vi "Read Peaks and Levels.vi"(0 "VISA resource name":refnum<visa-resource-name>, 5 "Enable Unbuffered Data (Enabled)":bool=TRUE, 11 "error in (no error)":errorcluster) -> (2 "Status":T2 {"Time Stamp" format="%#_20f"; "Operating Mode" items=["Stand-Alone", "Master", "End Slave", "Middle Slave"]; "Trigger Mode" items=["Untriggered", "Software Triggered", "Hardware Triggered"]; "Full Spectrum Radix" format="%b"}, 3 "Data Status":T3 {"Sub-Channel" items=["None", "1", "2", "3", "4"]; "Time Stamp" format="%#_20f"}, 4 "VISA resource name out":refnum<visa-resource-name>, 6 "Number of Sensors":u16[](array[numeric]), 8 "Amplitude (dBm)":i16[](array[numeric]), 10 "Peak Wavelengths (nm)":dbl[][](array[numeric]) format="%#_10g", 13 "Reserved":T1, 14 "Trigger Mode":u8(ring) items=["Untriggered", "Software Triggered", "Hardware Triggered"], 15 "error out":errorcluster)   [LabVIEW 2024, in "Micron Optics sm130.lvlib"]
doc: "Displays the peaks and levels. Peaks correspond to Peak Wavelengths in nm and Levels to Amplitudes in dBm."
uses:
  Micron Optics sm130.lvlib
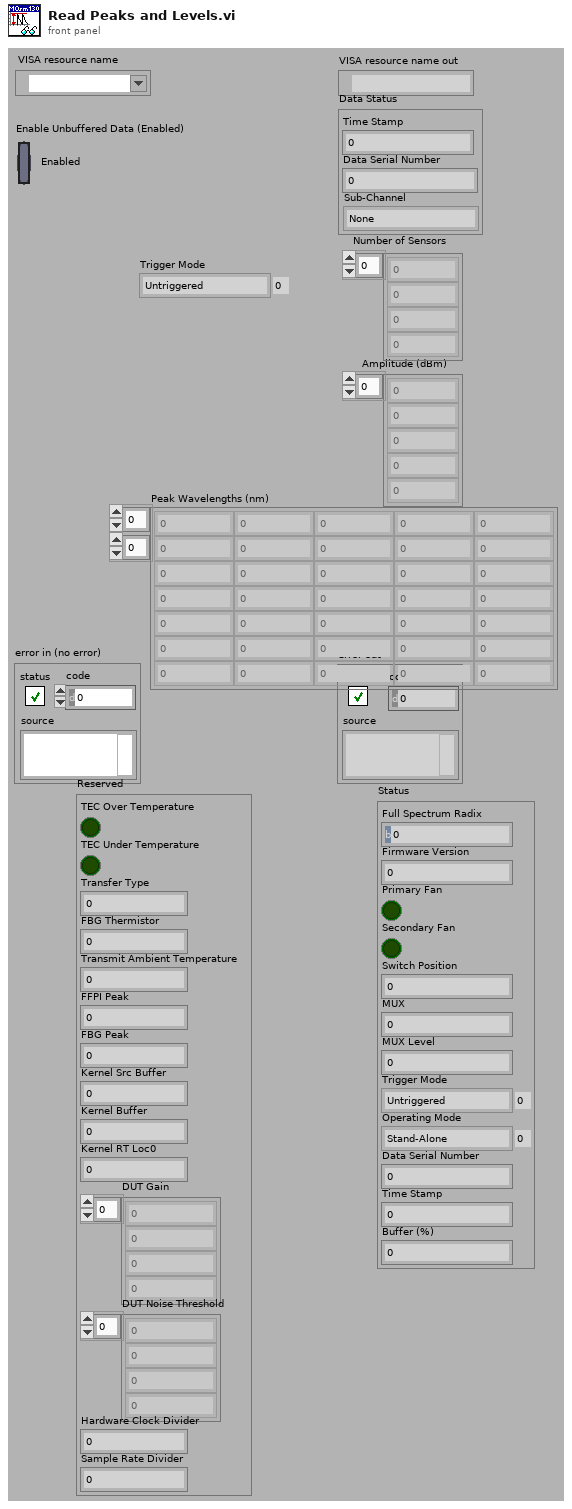
[diagram p1: front panel]
types:
  T1 = cluster{"Transmit Ambient Temperature":dbl, "FBG Thermistor":i16, "FFPI Peak":u16, "FBG Peak":dbl, "Kernel Src Buffer":u16, "Kernel Buffer":u16, "Kernel RT Loc0":u32, "DUT Gain":u16[], "DUT Noise Threshold":u16[], "Hardware Clock Divider":u16, "Sample Rate Divider":u16, "TEC Over Temperature":bool, "TEC Under Temperature":bool, "Transfer Type":u8}
  T2 = cluster{"Full Spectrum Radix":u8, "Firmware Version":u8, "Primary Fan":bool, "Secondary Fan":bool, "Switch Position":u8, "MUX":u8, "Trigger Mode":u8, "Operating Mode":u8, "Data Serial Number":u32, "Time Stamp":dbl, "Buffer (%)":u8, "MUX Level":u8}
  T3 = cluster{"Data Serial Number":u32, "Time Stamp":dbl, "Sub-Channel":u8}
  T4 = cluster{"Data Serial Number":u32, "Time Stamp":dbl, "Switch Position":u8}
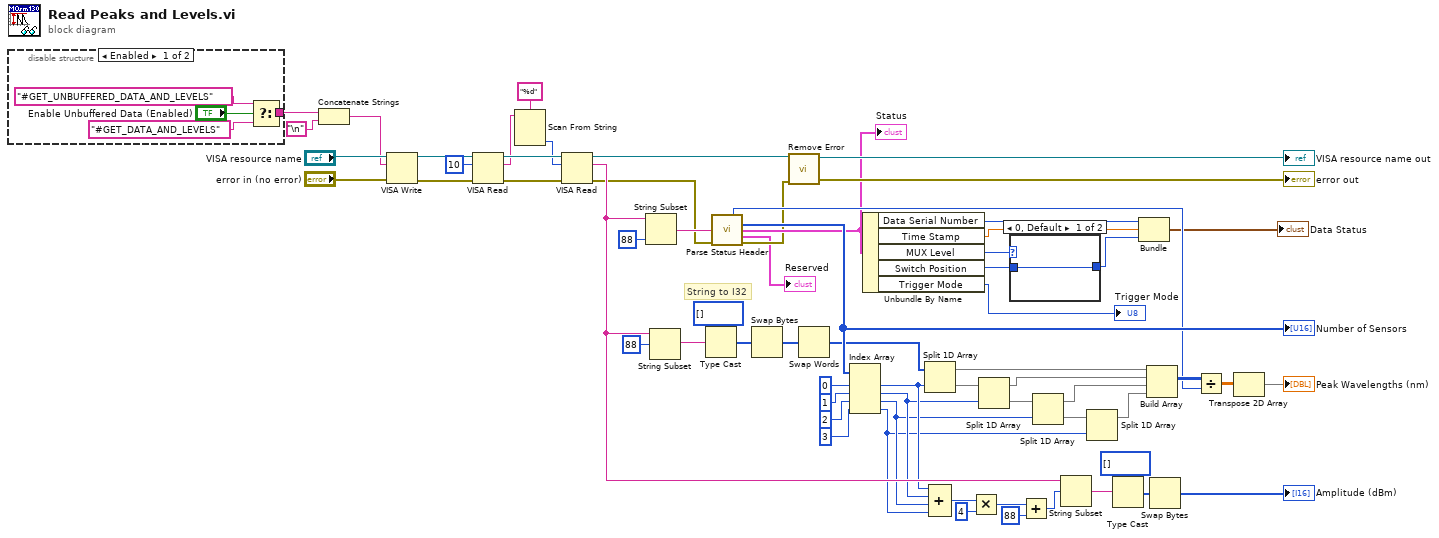
[diagram p0: block diagram]
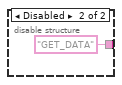
[diagram p2: hidden frame]
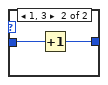
[diagram p3: hidden frame]
diagram:
  # "String to I32"
  n1 = disable-structure shown="Enabled" {
    disable-tunnel: [w66 "GET_DATA" ("f")] -> w4
    frame Enabled {
      n2 = Select(t="#GET_UNBUFFERED_DATA_AND_LEVELS" ("string"), s="Enable Unbuffered Data (Enabled)", f="#GET_DATA_AND_LEVELS") -> (s? t:f=w66:string)
    }
    frame Disabled {
    }
  }
  n3 = Concatenate Strings(w4, "\n") -> (w55:string)
  n4 = VISA Write(VISA resource name="VISA resource name", write buffer=w55, error in (no error)="error in (no error)") -> (VISA resource name out=w60:refnum<visa-resource-name>, error out=w59:errorcluster)  [unwired: 1 out]
  n5 = VISA Read(VISA resource name=w60, byte count=u32 10, error in (no error)=w59) -> (VISA resource name out=w65:refnum<visa-resource-name>, read buffer=w62:string, error out=w64:errorcluster)  [unwired: 1 out]
  n6 = Scan From String(format string="%d", input string=w62) -> (output 1=w61:i32)  [unwired: 3 in, 3 out]
  n7 = VISA Read(VISA resource name=w65, byte count=w61, error in (no error)=w64) -> (VISA resource name out=w54:refnum<visa-resource-name>, read buffer=w24:string, error out=w6:errorcluster)  [unwired: 1 out]
  n8 = String Subset(string=w24, length (rest)=88 ("length (rest)")) -> (substring=w50:string)  [unwired: 1 in]
  n9 = String Subset(string=w24, offset (0)=88 ("length (rest)")) -> (substring=w43:string)  [unwired: 1 in]
  n10 = Type Cast(type=i32[] [], x=w43) -> (*(type *) &x=w40:i32[])
  n11 = call "Parse Status Header.vi"("Status Header In"=w50, "error in (no error)"=w6) -> ("Granularity"=w30:u32, "Number of Sensors"=w48:u16[], "Status"=w13:T2, "Reserved"=→"Reserved":T1, "error out"=w5:errorcluster)  [unwired: 7 in, 2 out]
  "Number of Sensors" <- w48
  "Status" <- w13
  n12 = Swap Bytes(anything=w40) -> (byte swapped=w41:i32[])
  n13 = call "Remove Error.vi"("error in (no error)"=w5, "VISA resource name"=w54) -> ("error out"=→"error out":errorcluster, "VISA resource name out"=→"VISA resource name out":refnum<visa-resource-name>)  [unwired: 8 in]
  n14 = Swap Words(1:w41) -> (0:w39:i32[])
  n15 = Index Array(array=w48, index #1=0 ("index"), index #2=1 ("index"), index #3=2 ("index"), index #4=3 ("index")) -> (element #1=w22:u16, element #2=w21:u16, element #3=w20:u16, element #4=w19:u16)
  n16 = Unbundle By Name(w13) -> ("Data Serial Number"=w12:u32, "Time Stamp"=w11:dbl, "MUX Level"=w9:u8, "Switch Position"=w8:u8, "Trigger Mode"=→"Trigger Mode":u8)
  n17 = Split 1D Array(array=w39, index=w22) -> (first subarray=w35:i32[], second subarray=w38:i32[])
  n18 = Compound Arithmetic op=ADD(w22, w21, w20, w19) -> (w18:u16)
  n19 = Multiply(x=w18, y=u16 4) -> (x*y=w16:u16)
  n20 = Split 1D Array(array=w38, index=w21) -> (first subarray=w34:i32[], second subarray=w37:i32[])
  n21 = case shown="0, Default" w9 {
    tunnel: w8 -> [w71 w73]
    tunnel: [w71 w72] -> w7
    frame 0, Default {
    }
    frame 1, 3 {
      n22 = Increment(x=w73) -> (x+1=w72:u8)
    }
  }
  n23 = Add(x=w16, y=88) -> (x+y=w15:i32)
  n24 = Split 1D Array(array=w37, index=w20) -> (first subarray=w33:i32[], second subarray=w36:i32[])
  n25 = String Subset(string=w24, offset (0)=w15) -> (substring=w25:string)  [unwired: 1 in]
  n26 = Split 1D Array(array=w36, index=w19) -> (first subarray=w32:i32[])  [unwired: 1 out]
  n27 = Type Cast(type=i16[] [], x=w25) -> (*(type *) &x=w26:i16[])
  n28 = Bundle("Data Serial Number"=w12, "Time Stamp"=w11, "Switch Position"=w7) -> (→"Data Status":T4)  [unwired: 1 in]
  n29 = Build Array(w35, w34, w33, w32) -> (w31:i32[][])
  n30 = Swap Bytes(anything=w26) -> (byte swapped=→"Amplitude (dBm)":i16[])
  n31 = Divide(x=w31, y=w30) -> (x/y=w29:dbl[][])
  n32 = Transpose 2D Array(2D array=w29) -> (transposed array=→"Peak Wavelengths (nm)":dbl[][])
